vi "test_fgen.vi"() -> ()   [LabVIEW 2021]
uses:
  <vilib>/Platform/TimedLoop/XDataNode/timing_clust.ctl
  <vilib>/Platform/TimedLoop/XDataNode/nitl_modes.ctl
  <vilib>/Platform/TimedLoop/XDataNode/wakeup.ctl
  <vilib>/Platform/TimedLoop/XDataNode/XDataNode.xnode
  <vilib>/Analysis/NI_AALBase.lvlib
  <vilib>/Platform/TimedLoop/XDataNode/XDNodeRunTimeDep.lvlib
panel:
  in  "stop":bool
  in  "Tab Control":enum32{"Page 1", "Page 2"}(tab)
  out "Fgen Waveform":dbl[](graph)
  out "Analog Output Waveform":dbl(graph)
  in  "Amplitude":dbl=1.0 format="%0.2f"
  in  "Frequency":dbl=1.0 format="%0.2f"
  in  "dt (ms)":i64
  out "element":dbl
  out "Fgen Sinusoidal Pattern":dbl[](array[numeric])
  out "# cycles":dbl
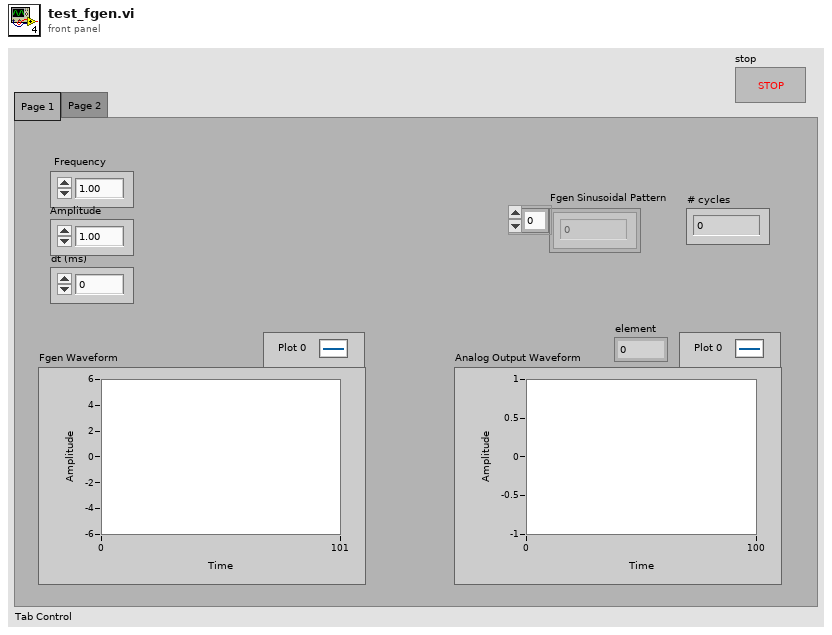
[diagram p1: front panel]
types:
  T1 = typedef "XDNodeRunTimeDep.lvlib/timing_clust.ctl" = cluster{"Expected End [f-1]":u64, "Actual End [f-1]":u64, "Finished Late? [f-1]":bool, "Expected End [i-1]":u64, "Actual End [i-1]":u64, "Finished Late? [i-1]":bool, "Expected Start [i]":u64, "Actual Start [i]":u64, "Expected Start [f]":u64, "Actual Start [f]":u64, "Source Name":string, "Structure Name":string, "Period":i64, "Deadline":i64, "Offset":i64, "Start":i64, "Priority":i32, "Timeout":i32, "Mode":T2, "Wakeup Reason":T3, "Error":errorcluster, "Source Type":string, "Secondary Source Type":string, "Global End Time":u64, "Global Start Time":u64, "Frame Duration":u64, "Iteration Duration":u64, "Assigned CPU":i32, "I/O Scan Engine Mode":u32}
  T2 = typedef "XDNodeRunTimeDep.lvlib/nitl_modes.ctl" = enum32{"No Change", "Process missed periods, maintain original phase", "Discard missed periods, maintain original phase", "Process missed periods, ignore original phase", "Discard missed periods, ignore original phase"}
  T3 = typedef "XDNodeRunTimeDep.lvlib/wakeup.ctl" = enum32{"Normal", "Aborted", "Asynchronous wakeup", "Timing source error", "Timed loop error", "Timeout"}
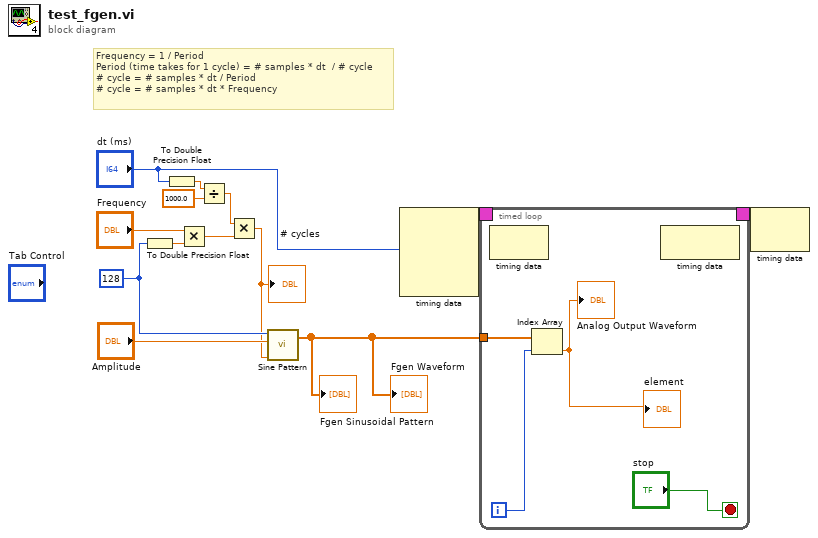
[diagram p0: block diagram]
diagram:
  w7 = 128 ("samples")
  # "Frequency = 1 / Period\nPeriod (time takes for 1 cycle) = # samples * dt  / # cycle\n# cycle = # samples * dt / Period\n# cycle = # samples * dt * Frequency"
  n1 = To Double Precision Float(number=w7) -> (double precision float=w8:dbl)
  n2 = To Double Precision Float(number="dt (ms)") -> (double precision float=w2:dbl)
  n3 = Multiply(x="Frequency", y=w8) -> (x*y=w6:dbl)
  n4 = Divide(x=w2, y=1000.0) -> (x/y=w1:dbl)
  n5 = Multiply(x=w1, y=w6) -> (x*y=w5:dbl)
  "# cycles" <- w5
  n6 = call <vilib>:"Sine Pattern.vi"("cycles"=w5, "amplitude"="Amplitude", "samples"=w7) -> ("Sinusoidal Pattern"=w10:dbl[])  [unwired: 1 in, 1 out]
  "Fgen Sinusoidal Pattern" <- w10
  "Fgen Waveform" <- w10
  n7 = node-c288("dt (ms)") -> (w13:T1)  [unwired: 3 in]
  n8 = timed-loop {
    timing: w13 -> [_]
    timing-out: [_] -> w12
    tunnel: w10 -> [w16]
    i -> [w17]
    stop <- "stop" stop-if-true
    n9 = node-c288() -> ()  [unwired: 1 in, 1 out]
    n10 = Index Array(array=w16, index=w17) -> (element=→"Analog Output Waveform" →"element":dbl)
    n11 = node-c288() -> ()  [unwired: 1 in, 1 out]
  }
  n12 = node-c288(w12) -> ()  [unwired: 1 out]
